vi "channal power.vi"() -> ()   [LabVIEW 2014]
uses:
  <instrlib>/Agilent E1963/Public/Configure/Measurement/Configure Measurement Trigger (Channel Power).vi
  <instrlib>/Agilent E1963/Public/Configure/Measurement/Configure Measurement (Channel Power).vi
  <instrlib>/Agilent E1963/Public/Data/Read Measurement (Channel Power).vi
  <instrlib>/Agilent E1963/Agilent E1963.lvlib
  <instrlib>/Agilent E1968/Agilent E1968.lvlib
panel:
  out "Connected?":bool
  in  "Maximum Time (10000 ms) 2":u32=10000
  in  "Downlink Channel (10700)":i32=10700
  out "Average RMSCubed":dbl
  out "Average Channel Power":dbl
  out "Integrity Indicator":u16(ring) items=["Normal"=0, "No Result Available"=1, "Measurement Timeout"=2, "Hardware Not Installed"=3, "Hardware Error"=4, "Over Range"=5, "Under Range"=6, "Burst Short"=7, "Trigger Early or Fall Early"=8, "Trigger Late or Rise Late"=9, "Signal Too Noisy"=10, "Sync Not Found"=11, "Oven Out of Range"=12, "Unidentified Error"=13, "PCM Full Scale Warning"=14, "Questionable Result for Phase 1 Mobile"=15, "Questionable Result"=16, "Can Not Correlate"=17, "Frequency Out of Range"=18, "Uncalibrated Due to Temperature"=19, "Potential Receiver Saturation"=20, "Parameter Error"=21, "Unsupported Configuration"=22, "Call Processing Operation Failed"=23, "Calibration Error"=24, "Burst Not Found"=25, "Missing Loopback Packets or AT Buffer Overflow"=26, "No AT Loopback Packets"=27, "Questionable MS-to-Cell Data"=28, "Trigger Missed"=30, "Dual Measurement Request"=31, "Measurement Not Licensed"=32]
  in  "Maximum Time (10000 ms)":u32=10000
  in  "Measurement Interval (6.667e-4 s)":dbl=0.0006667
  in  "Trigger Delay (0.0 s)":dbl format="%#_13g"
  in  "Trigger Source (4: Auto)":u16(ring)=4 items=["Immediate", "Protocol", "RF Rise", "External", "Auto", "HS-DPCCH"]
  in  "Measurement Type (0: All)":u16(ring) items=["All"=0, "AF Analyzer"=1, "Frequency Stability"=3, "HSDPA Block Error Ratio"=4, "Swept Audio"=5, "Spectrum Monitor"=6, "Adjacent Channel Leakage"=7, "Loopback Bit Error Ratio"=8, "Loopback Block Error Ratio"=9, "Code Domain"=10, "Channel Power"=11, "Dynamic Power Analysis"=12, "I/Q Tuning"=15, "Occupied Bandwidth"=16, "Spectrum Emission Mask"=19, "Thermal Power"=21, "Waveform Quality"=22]
  in  "VISA resource name":refnum<visa-resource-name>
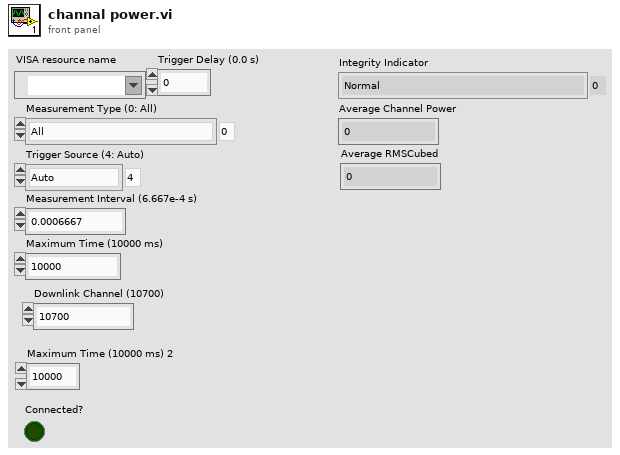
[diagram p1: front panel]
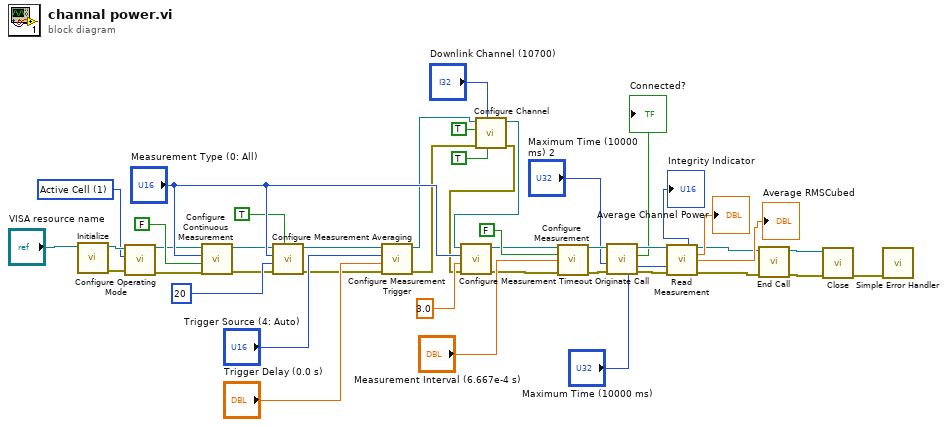
[diagram p0: block diagram]
diagram:
  w11 = u16 1 items=["Cell Off", "Active Cell", "FDD Test", "CW"] ("Operating Mode (1: Active Cell)")
  n1 = call <instrlib>:"Initialize.vi"("VISA resource name"="VISA resource name") -> ("error out"=w15:errorcluster, "VISA resource name out"=w12:refnum<visa-resource-name>)  [unwired: 9 in]
  n2 = call <instrlib>:"Configure Operating Mode.vi"("error in (no error)"=w15, "Operating Mode (1: Active Cell)"=w11, "VISA resource name"=w12) -> ("error out"=w14:errorcluster, "VISA resource name out"=w13:refnum<visa-resource-name>)  [unwired: 7 in]
  n3 = call <instrlib>:"Configure Continuous Measurement.vi"("error in (no error)"=w14, "Enable Continuous Arming (F:Disable)"=FALSE, "Measurement Type (0: All)"="Measurement Type (0: All)", "VISA resource name"=w13) -> ("error out"=w31:errorcluster, "VISA resource name out"=w30:refnum<visa-resource-name>)  [unwired: 6 in]
  n4 = call <instrlib>:"Configure Measurement Averaging.vi"("Enable Multi-measurement (F:Disable)"=TRUE, "error in (no error)"=w31, "Number of Measurements (10)"=20, "Measurement Type (1: AF Analyzer)"="Measurement Type (0: All)", "VISA resource name"=w30) -> ("error out"=w32:errorcluster, "VISA resource name out"=w29:refnum<visa-resource-name>)  [unwired: 5 in]
  n5 = call-poly <instrlib>:"Configure Measurement Trigger.vi"("error in (no error)"=w32, "Trigger Delay (0.0 s)"="Trigger Delay (0.0 s)", "Trigger Source (4: Auto)"="Trigger Source (4: Auto)", "VISA resource name"=w29) -> ("error out"=w17:errorcluster, "VISA resource name out"=w19:refnum<visa-resource-name>)  [unwired: 6 in]
  n6 = call <instrlib>:"Configure Channel.vi"("Enable Frequency Band Indicator (T:Enable)"=TRUE, "Downlink Channel (10700)"="Downlink Channel (10700)", "error in (no error)"=w17, "Auto Uplink Channel (T:Enable)"=TRUE, "VISA resource name"=w19) -> ("error out"=w16:errorcluster, "VISA resource name out"=w18:refnum<visa-resource-name>)  [unwired: 5 in]
  n7 = call <instrlib>:"Configure Measurement Timeout.vi"("error in (no error)"=w16, "Timeout (10.0 s)"=3.0, "Measurement Type (1: GSM Analog Audio)"="Measurement Type (0: All)", "VISA resource name"=w18) -> ("error out"=w34:errorcluster, "VISA resource name out"=w33:refnum<visa-resource-name>)  [unwired: 6 in]
  n8 = call-poly <instrlib>:"Configure Measurement.vi"("VISA resource name"=w33, "Enable RRC Filter (F:Disable)"=FALSE, "Measurement Interval (6.667e-4 s)"="Measurement Interval (6.667e-4 s)", "error in (no error)"=w34) -> ("VISA resource name out"=w9:refnum<visa-resource-name>, "error out"=w10:errorcluster)  [unwired: 10 in]
  n9 = call <instrlib>:"Originate Call.vi"("error in (no error)"=w10, "Maximum Time (10000 ms)"="Maximum Time (10000 ms) 2", "VISA resource name"=w9) -> ("error out"=w8:errorcluster, "Connected?"=→"Connected?":bool, "VISA resource name out"=w6:refnum<visa-resource-name>)  [unwired: 6 in]
  n10 = call-poly <instrlib>:"Read Measurement.vi"("VISA resource name"=w6, "Maximum Time (10000 ms)"="Maximum Time (10000 ms)", "error in (no error)"=w8) -> ("Integrity Indicator"=→"Integrity Indicator":u16, "VISA resource name out"=w4:refnum<visa-resource-name>, "Average Channel Power"=→"Average Channel Power":dbl, "Average RMSCubed"=→"Average RMSCubed":dbl, "error out"=w3:errorcluster)  [unwired: 8 in]
  n11 = call <instrlib>:"End Call.vi"("error in (no error)"=w3, "VISA resource name"=w4) -> ("error out"=w1:errorcluster, "VISA resource name out"=w2:refnum<visa-resource-name>)  [unwired: 8 in]
  n12 = call <instrlib>:"Close.vi"("error in (no error)"=w1, "VISA resource name"=w2) -> ("error out"=w25:errorcluster)  [unwired: 9 in]
  n13 = call <vilib>:"Simple Error Handler.vi"("error in (no error)"=w25) -> ()  [unwired: 4 in, 5 out]
